vi "Measurement.Uninit.vi"(8 "error in (no error)":errorcluster, 11 "Measurement.IVCurve in":refnum<class "Measurement.IVCurve.lvclass">) -> (0 "error out":errorcluster, 3 "Measurement.IVCurve out":refnum<class "Measurement.IVCurve.lvclass">)   [LabVIEW 2019, in "Measurement.IVCurve.lvclass"]
uses:
  Measurement.IVCurve.lvclass
  SMU/SMU.lvclass
  E:/UPWORK/Laser Tool/Laser/project/Subsystems/Device/Device.lvclass
  Device/Device.lvclass
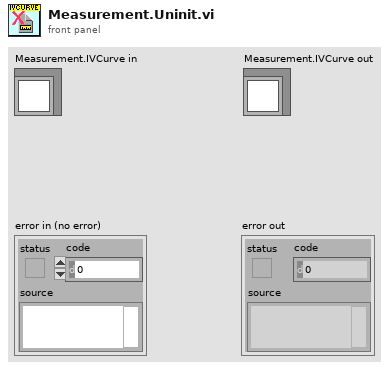
[diagram p1: front panel]
types:
  T1 = typedef "Measurement.IVCurve.lvclass/Dependencies--Cluster.ctl" = cluster{"SMU":refnum<class "SMU.lvclass">}
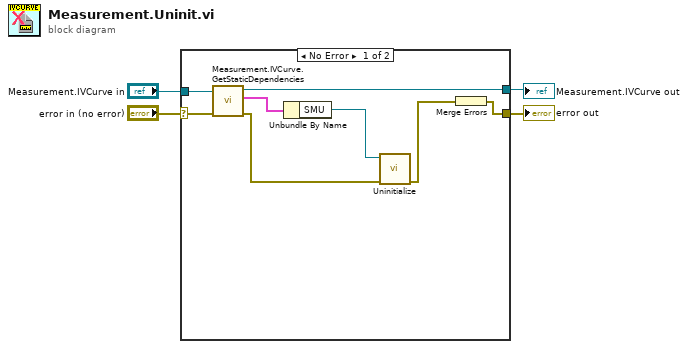
[diagram p0: block diagram]
diagram:
  n1 = case shown="No Error" "error in (no error)" {
    selector: "error in (no error)" -> [w11 w13]
    tunnel: "Measurement.IVCurve in" -> [w12 w14]
    tunnel: [w10 w14] -> w2
    tunnel: [w5 w13] -> w1
    frame No Error {
      n2 = call "Measurement.IVCurve.GetStaticDependencies.vi"("error in (no error)"=w11, "Measurement.IVCurve in"=w12) -> ("error out"=w7:errorcluster, "Dependencies"=w9:T1, "Measurement.IVCurve out"=w10:refnum<class "Measurement.IVCurve.lvclass">)  [unwired: 7 in]
      n3 = Unbundle By Name(w9) -> ("SMU"=w8:refnum<class "SMU.lvclass">)
      n4 = call "Uninitialize.vi"("error in (no error)"=w7, "Device in"=w8) -> ("error out"=w6:errorcluster)  [unwired: 8 in, 1 out]
      n5 = Merge Errors(w6) -> (w5:errorcluster)
    }
    frame Error {
    }
  }
  "error out" <- w1
  "Measurement.IVCurve out" <- w2
